vi "ReadPAQtags.vi"(8 "error in (no error)":errorcluster, 11 "DBAL-SQLite in":refnum<class "DBAL-SQLite.lvclass">) -> (0 "error out":errorcluster, 2 "PAQ_TAGs":T1 {"TAGprop"."TagFunc" format="%08x"; "TAGprop"."RangeL" format="%.2f"; "TAGprop"."RangeH" format="%.2f"}, 3 "DBAL-SQLite out":refnum<class "DBAL-SQLite.lvclass">)   [LabVIEW 2014, in "DBAL-SQLite.lvclass"]
doc: "Read the PAQ Qtype TAG properties from the database"
uses:
  DBAL-SQLite.lvclass
  controls/DBAL_TAGprops.ctl
  controls/DBAL_TAGpropEdit.ctl
  Common/controls/typedef_com_TagProp.ctl
  DBAL.lvclass
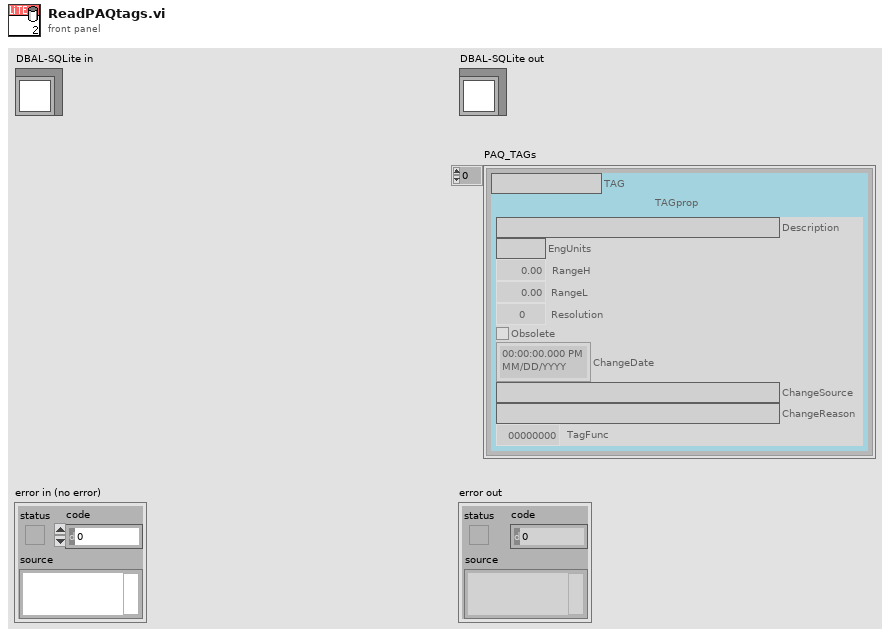
[diagram p1: front panel]
types:
  T1 = typedef "DBAL_TAGprops.ctl" = T2[]
  T2 = typedef "DBAL_TAGpropEdit.ctl" = cluster{"TAG":string, "TAGprop":T3}
  T3 = typedef "typedef_com_TagProp.ctl" = cluster{"Description":string, "EngUnits":string, "RangeH":dbl, "RangeL":dbl, "Resolution":i32, "Obsolete":bool, "ChangeDate":timestamp, "ChangeSource":string, "ChangeReason":string, "TagFunc":u32}
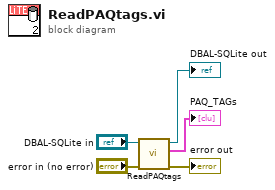
[diagram p0: block diagram]
diagram:
  n1 = call-parent "ReadPAQtags.vi"("error in (no error)"="error in (no error)", "DBAL in"="DBAL-SQLite in") -> ("error out"=→"error out":errorcluster, "PAQ_TAGs"=→"PAQ_TAGs":T1, "DBAL out"=→"DBAL-SQLite out":refnum<class "DBAL-SQLite.lvclass">)  [unwired: 7 in]
